vi "exportToDIAdem.vi"(11 "Export Data":string[][](array[string])) -> ()   [LabVIEW 2017]
doc: "This example uses the \"Register ActiveX Event Callback\" with a Microsoft Excel ActiveX control. \nIt demonstrates how to register an event and extract event data."
panel:
  out "Report Path Used":path
  out "Unique Temporary TDR File Path":path
  out "Unique Temporary TDMS File Path":path
  out "error out":errorcluster
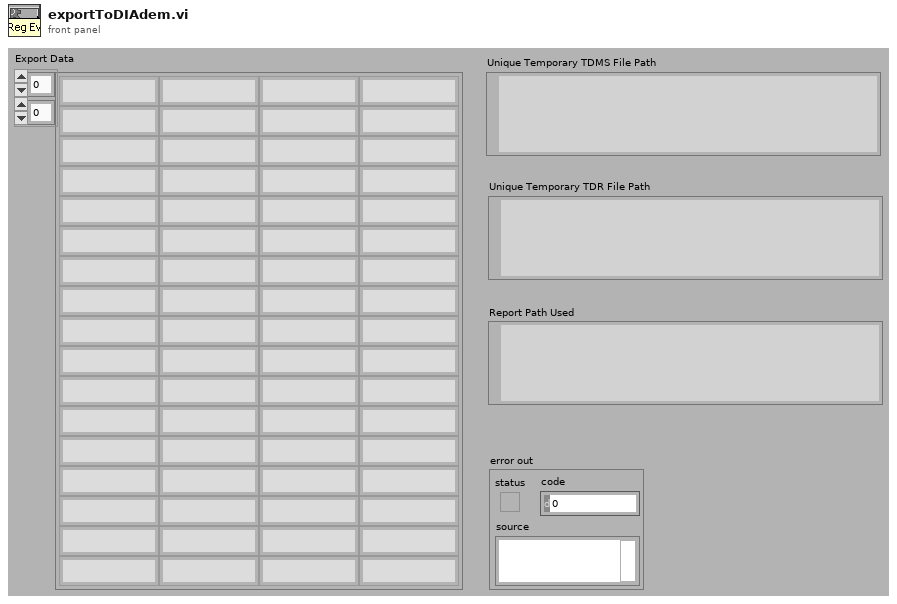
[diagram p1: front panel]
types:
  T1 = enum16{"open", "replace", "create", "open or create", "replace or create", "replace or create with confirmation"}
  T2 = enum16{"open", "open or create", "create or replace", "create", "open (read-only)"}
  T3 = enum32{"invalid app kind", "Development System", "Run Time System", "Student Edition", "Embedded LabVIEW", "Evaluation", "Custom"}
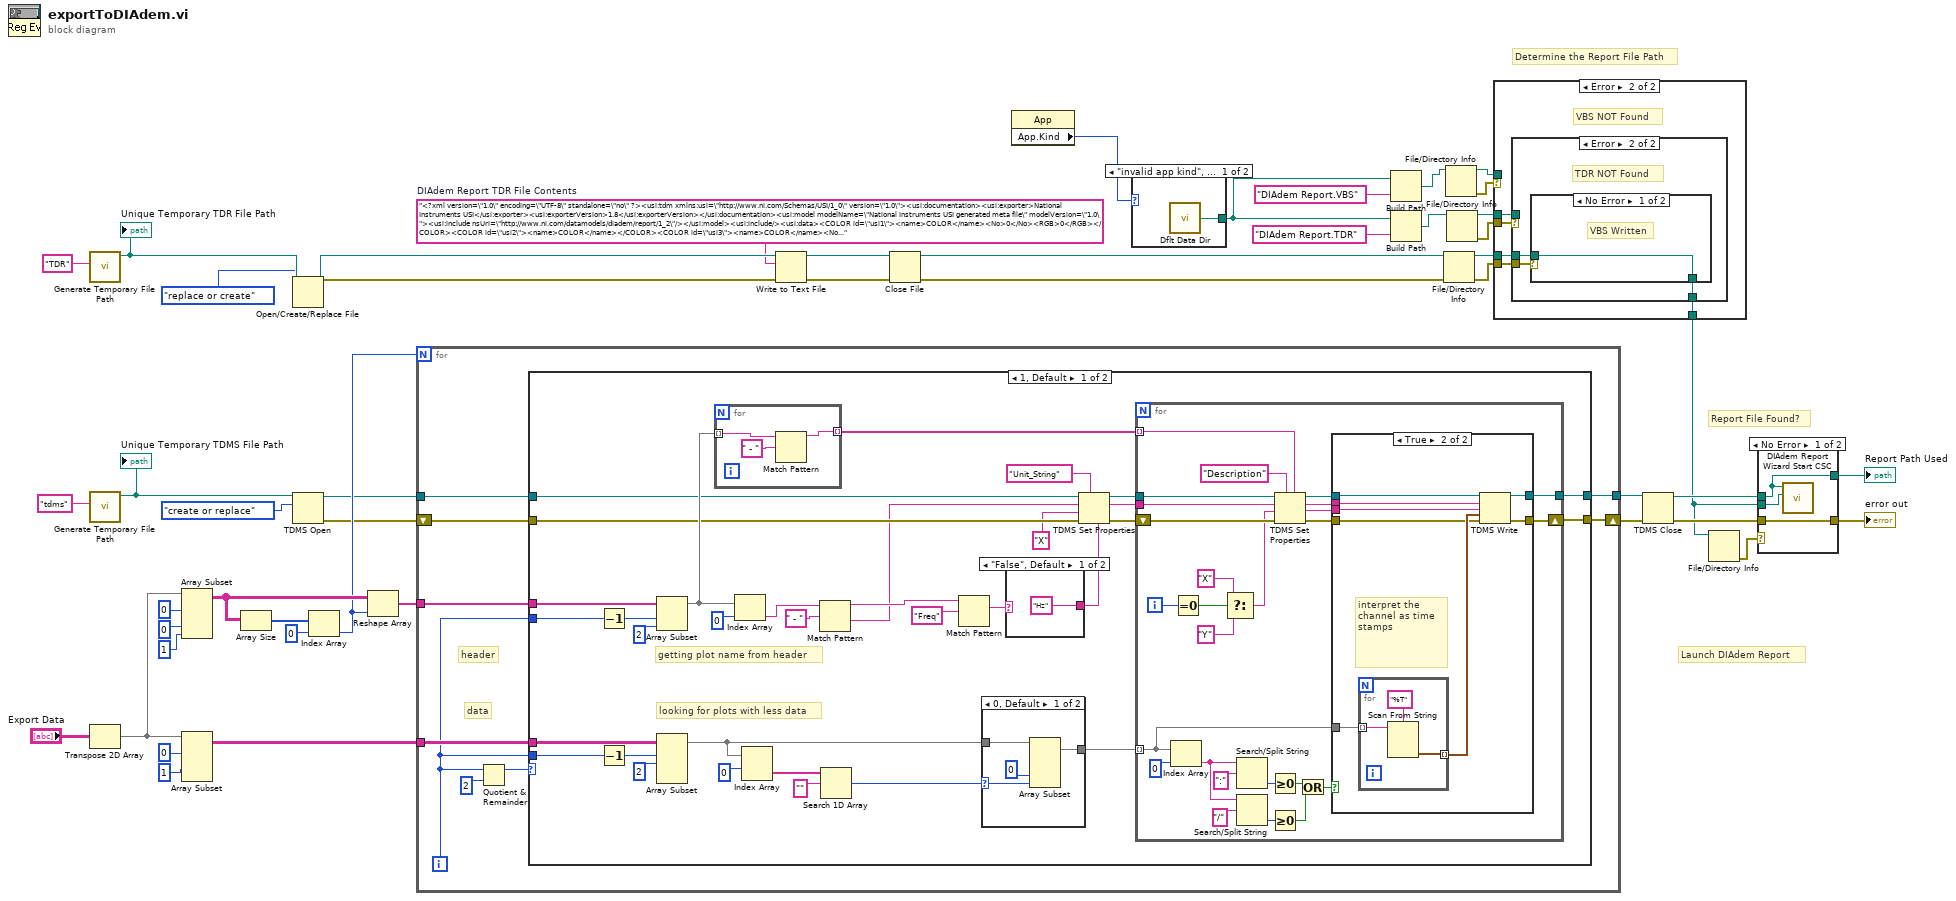
[diagram p0: block diagram]
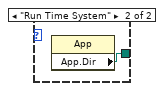
[diagram p2: hidden frame]
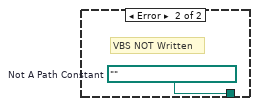
[diagram p5: hidden frame]
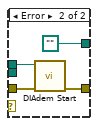
[diagram p6: hidden frame]
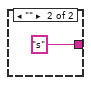
[diagram p7: hidden frame]
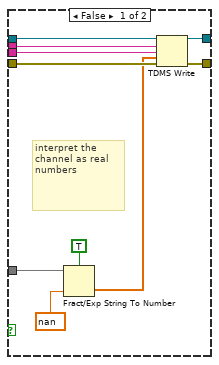
[diagram p8: hidden frame]
diagram:
  w15 = "<?xml version=\"1.0\" encoding=\"UTF-8\" standalone=\"no\" ?><usi:tdm xmlns:usi=\"http://www.ni.com/Schemas/USI/1_0\" version=\"1.0\"><usi:documentation><usi:exporter>National Instruments USI</usi:exporter><usi:exporterVersion>1.8</usi:exporterVersion></usi:documentation><usi:model modelName=\"National Instruments USI generated meta file\" modelVersion=\"1.0\"><usi:include nsUri=\"http://www.ni.com/datamodels/diadem/report/1_2\"/></usi:model><usi:include/><usi:data><COLOR id=\"usi1\"><name>COLOR</name><No>0</No><RGB>0</RGB></COLOR><COLOR id=\"usi2\"><name>COLOR</name></COLOR><COLOR id=\"usi3\"><name>COLOR</name><No>2</No></COLOR><COLOR id=\"usi4\"><name>COLOR</name><No>4</No><RGB>33554687</RGB></COLOR><COLOR id=\"usi5\"><name>COLOR</name><No>3</No><RGB>33619712</RGB></COLOR><COLOR id=\"usi6\"><name>COLOR</name><No>9</No><RGB>50266112</RGB></COLOR><COLOR id=\"usi7\"><name>COLOR</name><No>5</No><RGB>50266367</RGB></COLOR><COLOR id=\"usi8\"><name>COLOR</name><No>6</No><RGB>50331392</RGB></COLOR><COLOR id=\"usi9\"><name>COLOR</name><No>10</No><RGB>46186688</RGB></COLOR><COLOR id=\"usi10\"><name>COLOR</name><No>15</No><RGB>33619967</RGB></COLOR><COLOR id=\"usi11\"><name>COLOR</name><No>9</No><RGB>33554560</RGB></COLOR><COLOR id=\"usi12\"><name>COLOR</name><No>10</No><RGB>33587200</RGB></COLOR><COLOR id=\"usi13\"><name>COLOR</name></COLOR><COLOR id=\"usi14\"><name>COLOR</name></COLOR><COLOR id=\"usi15\"><name>COLOR</name></COLOR><COLOR id=\"usi16\"><name>COLOR</name><No>0</No><RGB>14737616</RGB><RGB2>15263976</RGB2></COLOR><COLOR id=\"usi17\"><name>COLOR</name></COLOR><COLOR id=\"usi18\"><name>COLOR</name></COLOR><COLOR id=\"usi19\"><name>COLOR</name></COLOR><COLOR id=\"usi20\"><name>COLOR</name></COLOR><COLOR id=\"usi21\"><name>COLOR</name></COLOR><COLOR id=\"usi22\"><name>COLOR</name></COLOR><COLOR id=\"usi23\"><name>COLOR</name></COLOR><COLOR id=\"usi24\"><name>COLOR</name></COLOR><COLOR id=\"usi25\"><name>COLOR</name></COLOR><COLOR id=\"usi26\"><name>COLOR</name></COLOR><COLOR id=\"usi27\"><name>COLOR</name></COLOR><COLOR id=\"usi28\"><name>COLOR</name></COLOR><COLOR id=\"usi29\"><name>COLOR</name></COLOR><COLOR id=\"usi30\"><name>COLOR</name><No>2</No><RGB>33554687</RGB></COLOR><COLOR id=\"usi31\"><name>COLOR</name><No>0</No><RGB>50331647</RGB><RGB2>15263976</RGB2></COLOR><COLOR id=\"usi32\"><name>COLOR</name><No>0</No><RGB>0</RGB><RGB2>0</RGB2><FillMode>Horizontal</FillMode></COLOR><COLOR id=\"usi33\"><name>COLOR</name><No>0</No><RGB>0</RGB><RGB2>0</RGB2><FillMode>Horizontal</FillMode></COLOR><COLOR id=\"usi34\"><name>COLOR</name><No>16</No><RGB>50331647</RGB></COLOR><COLOR id=\"usi35\"><name>COLOR</name></COLOR><COLOR id=\"usi36\"><name>COLOR</name><No>0</No><RGB>50331647</RGB></COLOR><COLOR id=\"usi37\"><name>COLOR</name></COLOR><COLOR id=\"usi38\"><name>COLOR</name></COLOR><COLOR id=\"usi39\"><name>COLOR</name></COLOR><COLOR id=\"usi40\"><name>COLOR</name></COLOR><COLOR id=\"usi41\"><name>COLOR</name></COLOR><COLOR id=\"usi42\"><name>COLOR</name><No>7</No><RGB>46186688</RGB></COLOR><COLOR id=\"usi43\"><name>COLOR</name><No>7</No><RGB>46186688</RGB></COLOR><COLOR id=\"usi44\"><name>COLOR</name><No>7</No><RGB>46186688</RGB></COLOR><COLOR id=\"usi45\"><name>COLOR</name><No>7</No><RGB>46186688</RGB></COLOR><COLOR id=\"usi46\"><name>COLOR</name><No>7</No><RGB>46186688</RGB></COLOR><COLOR id=\"usi47\"><name>COLOR</name><No>7</No><RGB>46186688</RGB></COLOR><COLOR id=\"usi48\"><name>COLOR</name><No>7</No><RGB>46186688</RGB></COLOR><COLOR id=\"usi49\"><name>COLOR</name><No>7</No><RGB>46186688</RGB></COLOR><COLOR id=\"usi50\"><name>COLOR</name><No>7</No><RGB>46186688</RGB></COLOR><COLOR id=\"usi51\"><name>COLOR</name><No>7</No><RGB>46186688</RGB></COLOR><COLOR id=\"usi52\"><name>COLOR</name><No>7</No><RGB>46186688</RGB></COLOR><COLOR id=\"usi53\"><name>COLOR</name><No>7</No><RGB>46186688</RGB></COLOR><COLOR id=\"usi54\"><name>COLOR</name><No>7</No><RGB>46186688</RGB></COLOR><COLOR id=\"usi55\"><name>COLOR</name><No>7</No><RGB>46186688</RGB></COLOR><COLOR id=\"usi56\"><name>COLOR</name><No>7</No><RGB>46186688</RGB></COLOR><COLOR id=\"usi57\"><name>COLOR</name><No>7</No><RGB>46186688</RGB></COLOR><COLOR id=\"usi58\"><name>COLOR</name><No>7</No><RGB>46186688</RGB></COLOR><COLOR id=\"usi59\"><name>COLOR</name><No>7</No><RGB>46186688</RGB></COLOR><COLOR id=\"usi60\"><name>COLOR</name><No>7</No><RGB>46186688</RGB></COLOR><COLOR id=\"usi61\"><name>COLOR</name><No>7</No><RGB>46186688</RGB></COLOR><COLOR id=\"usi62\"><name>COLOR</name><RGB>50266112</RGB></COLOR><COLOR id=\"usi63\"><name>COLOR</name></COLOR><COLOR id=\"usi64\"><name>COLOR</name><RGB>50266112</RGB></COLOR><COLOR id=\"usi65\"><name>COLOR</name></COLOR><COLOR id=\"usi66\"><name>COLOR</name><No>2</No><RGB>33554687</RGB></COLOR><COLOR id=\"usi67\"><name>COLOR</name><No>4</No><RGB>50266112</RGB></COLOR><COLOR id=\"usi68\"><name>COLOR</name><No>4</No><RGB>50266112</RGB></COLOR><COLOR id=\"usi69\"><name>COLOR</name><No>2</No><RGB>33554687</RGB></COLOR><COLOR id=\"usi70\"><name>COLOR</name></COLOR><COLOR id=\"usi71\"><name>COLOR</name><No>2</No><RGB>33554687</RGB></COLOR><COLOR id=\"usi72\"><name>COLOR</name></COLOR><COLOR id=\"usi73\"><name>COLOR</name><No>2</No><RGB>33554687</RGB></COLOR><COLOR id=\"usi74\"><name>COLOR</name><No>3</No><RGB>33619712</RGB></COLOR><COLOR id=\"usi75\"><name>COLOR</name><No>4</No><RGB>50266112</RGB></COLOR><COLOR id=\"usi76\"><name>COLOR</name><No>5</No><RGB>50266367</RGB></COLOR><COLOR id=\"usi77\"><name>COLOR</name><No>6</No><RGB>50331392</RGB></COLOR><COLOR id=\"usi78\"><name>COLOR</name><No>7</No><RGB>46186688</RGB></COLOR><COLOR id=\"usi79\"><name>COLOR</name><No>8</No><RGB>33619967</RGB></COLOR><COLOR id=\"usi80\"><name>COLOR</name><No>9</No><RGB>33554560</RGB></COLOR><COLOR id=\"usi81\"><name>COLOR</name><No>10</No><RGB>33587200</RGB></COLOR><COLOR id=\"usi82\"><name>COLOR</name><No>11</No><RGB>41943040</RGB></COLOR><COLOR id=\"usi83\"><name>COLOR</name><No>12</No><RGB>41943168</RGB></COLOR><COLOR id=\"usi84\"><name>COLOR</name><No>13</No><RGB>41975808</RGB></COLOR><COLOR id=\"usi85\"><name>COLOR</name><No>14</No><RGB>41975936</RGB></COLOR><COLOR id=\"usi86\"><name>COLOR</name><No>15</No><RGB>33587328</RGB></COLOR><COLOR id=\"usi87\"><name>COLOR</name><No>4</No><RGB>50266112</RGB></COLOR><COLOR id=\"usi88\"><name>COLOR</name><No>4</No><RGB>50266112</RGB></COLOR><COLOR id=\"usi89\"><name>COLOR</name><No>4</No><RGB>50266112</RGB></COLOR><COLOR id=\"usi90\"><name>COLOR</name><No>4</No><RGB>50266112</RGB></COLOR><LINE id=\"usi91\"><name>FrameLine</name><Width>4</Width><Color>#xpointer(id(\"usi2\"))</Color></LINE><LINE id=\"usi92\"><name>LINE</name><Interval>2</Interval><Width>3</Width><Color>#xpointer(id(\"usi13\"))</Color></LINE><LINE id=\"usi93\"><name>LINE</name><Interval>2</Interval><Width>3</Width><Color>#xpointer(id(\"usi14\"))</Color></LINE><LINE id=\"usi94\"><name>LINE</name><Interval>2</Interval><Width>3</Width><Color>#xpointer(id(\"usi15\"))</Color></LINE><LINE id=\"usi95\"><name>LINE</name><Width>3</Width><Color>#xpointer(id(\"usi27\"))</Color></LINE><LINE id=\"usi96\"><name>LINE</name><Width>3</Width><Color>#xpointer(id(\"usi28\"))</Color></LINE><LINE id=\"usi97\"><name>LINE</name><Width>3</Width><Color>#xpointer(id(\"usi29\"))</Color></LINE><LINE id=\"usi98\"><name>LINE</name><Interval>2</Interval><Width>0</Width><Color>#xpointer(id(\"usi38\"))</Color></LINE><LINE id=\"usi99\"><name>LINE</name><Interval>2</Interval><Width>0</Width><Color>#xpointer(id(\"usi39\"))</Color></LINE><LINE id=\"usi100\"><name>LINE</name><Interval>2</Interval><Width>0</Width><Color>#xpointer(id(\"usi40\"))</Color></LINE><LINE id=\"usi101\"><name>LINE</name><Interval>2</Interval><Width>0</Width><Color>#xpointer(id(\"usi41\"))</Color></LINE><LINE id=\"usi102\"><name>LINE</name><Width>0</Width><Color>#xpointer(id(\"usi67\"))</Color></LINE><FONT id=\"usi103\"><name>FONT</name><Size>3</Size><PitchAndFamily>32</PitchAndFamily><Color>#xpointer(id(\"usi62\"))</Color></FONT><FONT id=\"usi104\"><name>FONT</name><Size>4</Size><PitchAndFamily>16</PitchAndFamily><Color>#xpointer(id(\"usi63\"))</Color></FONT><FONT id=\"usi105\"><name>FONT</name><Size>3</Size><PitchAndFamily>32</PitchAndFamily><Color>#xpointer(id(\"usi64\"))</Color></FONT><FONT id=\"usi106\"><name>FONT</name><Size>4</Size><Angle>90</Angle><PitchAndFamily>16</PitchAndFamily><Color>#xpointer(id(\"usi65\"))</Color></FONT><FONT id=\"usi107\"><name>FONT</name><FaceName>Times New Roman</FaceName><Size>4</Size><PitchAndFamily>16</PitchAndFamily><Color>#xpointer(id(\"usi68\"))</Color></FONT><FONT id=\"usi108\"><name>FONT</name><FaceName>Times New Roman</FaceName><Size>4</Size><PitchAndFamily>16</PitchAndFamily><Color>#xpointer(id(\"usi71\"))</Color></FONT><FONT id=\"usi109\"><name>FONT</name><Size>3</Size><PitchAndFamily>32</PitchAndFamily><Color>#xpointer(id(\"usi87\"))</Color></FONT><FONT id=\"usi110\"><name>FONT</name><Size>3</Size><PitchAndFamily>32</PitchAndFamily><Color>#xpointer(id(\"usi88\"))</Color></FONT><FONT id=\"usi111\"><name>FONT</name><FaceName>Arial</FaceName><Size>3</Size><PitchAndFamily>32</PitchAndFamily><Color>#xpointer(id(\"usi89\"))</Color></FONT><FONT id=\"usi112\"><name>FONT</name><FaceName>Arial</FaceName><Size>3</Size><PitchAndFamily>32</PitchAndFamily><Color>#xpointer(id(\"usi90\"))</Color></FONT><PALETTE2D id=\"usi113\"><Line>#xpointer(id(\"usi213\") id(\"usi214\") id(\"usi215\") id(\"usi216\") id(\"usi217\") id(\"usi218\") id(\"usi219\") id(\"usi220\") id(\"usi221\") id(\"usi222\") id(\"usi223\") id(\"usi224\") id(\"usi225\") id(\"usi226\") id(\"usi227\"))</Line></PALETTE2D><GLOBPAL id=\"usi114\"><name>global Palette 1</name><No>64</No><CtrlColorHSI>7925920 7925760</CtrlColorHSI><Line>#xpointer(id(\"usi92\"))</Line></GLOBPAL><GLOBPAL id=\"usi115\"><name>global Palette 2</name><No>64</No><CtrlColorHSI>7925920 7925999</CtrlColorHSI><Line>#xpointer(id(\"usi93\"))</Line></GLOBPAL><GLOBPAL id=\"usi116\"><name>global Palette 3</name><No>64</No><CtrlColorHSI>11858080 11857920</CtrlColorHSI><Line>#xpointer(id(\"usi94\"))</Line></GLOBPAL><CHANNEL id=\"usi117\"><name>TickChn</name></CHANNEL><CHANNEL id=\"usi118\"><name>TickChn</name></CHANNEL><CHANNEL id=\"usi119\"><name>XChn</name><No>1</No><ChnName>X</ChnName></CHANNEL><CHANNEL id=\"usi120\"><name>YChn</name><No>2</No><ChnName>Y</ChnName></CHANNEL><CHANNEL id=\"usi121\"><name>Y1Chn</name></CHANNEL><CHANNEL id=\"usi122\"><name>CHANNEL</name></CHANNEL><CHANNEL id=\"usi123\"><name>IndexChannel</name></CHANNEL><CHANNEL id=\"usi124\"><name>XChn</name></CHANNEL><CHANNEL id=\"usi125\"><name>YChn</name></CHANNEL><CHANNEL id=\"usi126\"><name>XChn</name></CHANNEL><CHANNEL id=\"usi127\"><name>YChn</name></CHANNEL><CHANNEL id=\"usi128\"><name>XChn</name></CHANNEL><CHANNEL id=\"usi129\"><name>YChn</name></CHANNEL><CHANNEL id=\"usi130\"><name>XChn</name></CHANNEL><CHANNEL id=\"usi131\"><name>YChn</name></CHANNEL><CHANNEL id=\"usi132\"><name>XChn</name></CHANNEL><CHANNEL id=\"usi133\"><name>YChn</name></CHANNEL><CHANNEL id=\"usi134\"><name>XChn</name></CHANNEL><CHANNEL id=\"usi135\"><name>YChn</name></CHANNEL><CHANNEL id=\"usi136\"><name>XChn</name></CHANNEL><CHANNEL id=\"usi137\"><name>YChn</name></CHANNEL><CHANNEL id=\"usi138\"><name>XChn</name></CHANNEL><CHANNEL id=\"usi139\"><name>YChn</name></CHANNEL><CHANNEL id=\"usi140\"><name>XChn</name></CHANNEL><CHANNEL id=\"usi141\"><name>YChn</name></CHANNEL><CHANNEL id=\"usi142\"><name>XChn</name></CHANNEL><CHANNEL id=\"usi143\"><name>YChn</name></CHANNEL><CHANNEL id=\"usi144\"><name>XChn</name></CHANNEL><CHANNEL id=\"usi145\"><name>YChn</name></CHANNEL><CHANNEL id=\"usi146\"><name>XChn</name></CHANNEL><CHANNEL id=\"usi147\"><name>YChn</name></CHANNEL><CHANNEL id=\"usi148\"><name>XChn</name></CHANNEL><CHANNEL id=\"usi149\"><name>YChn</name></CHANNEL><CHANNEL id=\"usi150\"><name>XChn</name></CHANNEL><CHANNEL id=\"usi151\"><name>YChn</name></CHANNEL><CHANNEL id=\"usi152\"><name>XChn</name></CHANNEL><CHANNEL id=\"usi153\"><name>YChn</name></CHANNEL><CHANNEL id=\"usi154\"><name>XChn</name></CHANNEL><CHANNEL id=\"usi155\"><name>YChn</name></CHANNEL><CHANNEL id=\"usi156\"><name>XChn</name></CHANNEL><CHANNEL id=\"usi157\"><name>YChn</name></CHANNEL><CHANNEL id=\"usi158\"><name>XChn</name></CHANNEL><CHANNEL id=\"usi159\"><name>YChn</name></CHANNEL><CHANNEL id=\"usi160\"><name>XChn</name></CHANNEL><CHANNEL id=\"usi161\"><name>YChn</name></CHANNEL><CHANNEL id=\"usi162\"><name>XChn</name></CHANNEL><CHANNEL id=\"usi163\"><name>YChn</name></CHANNEL><CHANNEL id=\"usi164\"><name>PositiveErrorChn</name></CHANNEL><CHANNEL id=\"usi165\"><name>NegativeErrorChn</name></CHANNEL><CHANNEL id=\"usi166\"><name>PositiveErrorChn</name></CHANNEL><CHANNEL id=\"usi167\"><name>NegativeErrorChn</name></CHANNEL><NUMERICLABEL id=\"usi168\"><name>NUMERICLABEL</name><RelPos>bottom</RelPos><Font>#xpointer(id(\"usi103\"))</Font></NUMERICLABEL><NUMERICLABEL id=\"usi169\"><name>NUMERICLABEL</name><RelPos>left</RelPos><Font>#xpointer(id(\"usi105\"))</Font></NUMERICLABEL><FREELABEL id=\"usi170\"><name>FREELABEL</name><Text>@@ChnComment(CurrChnNo)@@ [@@ChnDim(CurrChnNo)@@]</Text><DeltaX>100</DeltaX><DeltaY>-8.07</DeltaY><Font>#xpointer(id(\"usi104\"))</Font></FREELABEL><FREELABEL id=\"usi171\"><name>FREELABEL</name><Text>@@ChnComment(CurrChnNo)@@</Text><DeltaX>-7.51</DeltaX><DeltaY>100</DeltaY><Font>#xpointer(id(\"usi106\"))</Font></FREELABEL><AXISGROUP id=\"usi172\"><name>AxisGroup1</name><XAxis>#xpointer(id(\"usi228\"))</XAxis><YAxis>#xpointer(id(\"usi229\"))</YAxis><AXIS2D>#xpointer(id(\"usi230\"))</AXIS2D></AXISGROUP><PAGE id=\"usi173\"><name>Export From LabVIEW</name><Ratio>0.77</Ratio><Width>10</Width><Height>7.5</Height><PicDefExpand>1</PicDefExpand><Line>#xpointer(id(\"usi91\"))</Line><BackColor>#xpointer(id(\"usi1\"))</BackColor><ExpList>#xpointer(id(\"usi174\"))</ExpList><PalGlob>#xpointer(id(\"usi114\") id(\"usi115\") id(\"usi116\"))</PalGlob><Objects>#xpointer(id(\"usi230\"))</Objects><REPORT>#xpointer(id(\"usi175\"))</REPORT></PAGE><EXPANDLIST id=\"usi174\"><ExpListUse>1</ExpListUse><LineTypUse>0</LineTypUse><LineIntUse>0</LineIntUse><ExpListNo>8</ExpListNo><Line>#xpointer(id(\"usi231\") id(\"usi232\") id(\"usi233\") id(\"usi234\") id(\"usi235\") id(\"usi236\") id(\"usi237\") id(\"usi238\") id(\"usi239\") id(\"usi240\"))</Line></EXPANDLIST><REPORT id=\"usi175\"><name>lvtemporary_550384</name><LastName>lvtemporary_550384</LastName><ScaleNorm>0</ScaleNorm><BinaryRasterOps>13</BinaryRasterOps><Ratio>0.77</Ratio><Width>10</Width><Height>7.5</Height><Pages>#xpointer(id(\"usi173\"))</Pages></REPORT><AXISSYSTEM id=\"usi176\"><FrameDisplay>Frame</FrameDisplay><BackColor>#xpointer(id(\"usi16\"))</BackColor><FrameLine>#xpointer(id(\"usi95\"))</FrameLine><DisplayXAxis>#xpointer(id(\"usi177\"))</DisplayXAxis><DisplayYAxis>#xpointer(id(\"usi178\"))</DisplayYAxis><Sections>#xpointer(id(\"usi179\"))</Sections></AXISSYSTEM><DISPLAYAXIS id=\"usi177\"><GridLine>#xpointer(id(\"usi98\"))</GridLine><MiniTickLine>#xpointer(id(\"usi99\"))</MiniTickLine></DISPLAYAXIS><DISPLAYAXIS id=\"usi178\"><GridLine>#xpointer(id(\"usi100\"))</GridLine><MiniTickLine>#xpointer(id(\"usi101\"))</MiniTickLine></DISPLAYAXIS><SECTIONS id=\"usi179\"><name>Sections</name><Section>#xpointer(id(\"usi180\") id(\"usi181\") id(\"usi182\") id(\"usi183\") id(\"usi184\") id(\"usi185\") id(\"usi186\") id(\"usi187\") id(\"usi188\") id(\"usi189\") id(\"usi190\") id(\"usi191\") id(\"usi192\") id(\"usi193\") id(\"usi194\") id(\"usi195\") id(\"usi196\") id(\"usi197\") id(\"usi198\") id(\"usi199\"))</Section></SECTIONS><SECTION id=\"usi180\"><name>Section1</name><Color>#xpointer(id(\"usi42\"))</Color><XChn>#xpointer(id(\"usi124\"))</XChn><YChn>#xpointer(id(\"usi125\"))</YChn></SECTION><SECTION id=\"usi181\"><name>Section2</name><Color>#xpointer(id(\"usi43\"))</Color><XChn>#xpointer(id(\"usi126\"))</XChn><YChn>#xpointer(id(\"usi127\"))</YChn></SECTION><SECTION id=\"usi182\"><name>Section3</name><Color>#xpointer(id(\"usi44\"))</Color><XChn>#xpointer(id(\"usi128\"))</XChn><YChn>#xpointer(id(\"usi129\"))</YChn></SECTION><SECTION id=\"usi183\"><name>Section4</name><Color>#xpointer(id(\"usi45\"))</Color><XChn>#xpointer(id(\"usi130\"))</XChn><YChn>#xpointer(id(\"usi131\"))</YChn></SECTION><SECTION id=\"usi184\"><name>Section5</name><Color>#xpointer(id(\"usi46\"))</Color><XChn>#xpointer(id(\"usi132\"))</XChn><YChn>#xpointer(id(\"usi133\"))</YChn></SECTION><SECTION id=\"usi185\"><name>Section6</name><Color>#xpointer(id(\"usi47\"))</Color><XChn>#xpointer(id(\"usi134\"))</XChn><YChn>#xpointer(id(\"usi135\"))</YChn></SECTION><SECTION id=\"usi186\"><name>Section7</name><Color>#xpointer(id(\"usi48\"))</Color><XChn>#xpointer(id(\"usi136\"))</XChn><YChn>#xpointer(id(\"usi137\"))</YChn></SECTION><SECTION id=\"usi187\"><name>Section8</name><Color>#xpointer(id(\"usi49\"))</Color><XChn>#xpointer(id(\"usi138\"))</XChn><YChn>#xpointer(id(\"usi139\"))</YChn></SECTION><SECTION id=\"usi188\"><name>Section9</name><Color>#xpointer(id(\"usi50\"))</Color><XChn>#xpointer(id(\"usi140\"))</XChn><YChn>#xpointer(id(\"usi141\"))</YChn></SECTION><SECTION id=\"usi189\"><name>Section10</name><Color>#xpointer(id(\"usi51\"))</Color><XChn>#xpointer(id(\"usi142\"))</XChn><YChn>#xpointer(id(\"usi143\"))</YChn></SECTION><SECTION id=\"usi190\"><name>Section11</name><Color>#xpointer(id(\"usi52\"))</Color><XChn>#xpointer(id(\"usi144\"))</XChn><YChn>#xpointer(id(\"usi145\"))</YChn></SECTION><SECTION id=\"usi191\"><name>Section12</name><Color>#xpointer(id(\"usi53\"))</Color><XChn>#xpointer(id(\"usi146\"))</XChn><YChn>#xpointer(id(\"usi147\"))</YChn></SECTION><SECTION id=\"usi192\"><name>Section13</name><Color>#xpointer(id(\"usi54\"))</Color><XChn>#xpointer(id(\"usi148\"))</XChn><YChn>#xpointer(id(\"usi149\"))</YChn></SECTION><SECTION id=\"usi193\"><name>Section14</name><Color>#xpointer(id(\"usi55\"))</Color><XChn>#xpointer(id(\"usi150\"))</XChn><YChn>#xpointer(id(\"usi151\"))</YChn></SECTION><SECTION id=\"usi194\"><name>Section15</name><Color>#xpointer(id(\"usi56\"))</Color><XChn>#xpointer(id(\"usi152\"))</XChn><YChn>#xpointer(id(\"usi153\"))</YChn></SECTION><SECTION id=\"usi195\"><name>Section16</name><Color>#xpointer(id(\"usi57\"))</Color><XChn>#xpointer(id(\"usi154\"))</XChn><YChn>#xpointer(id(\"usi155\"))</YChn></SECTION><SECTION id=\"usi196\"><name>Section17</name><Color>#xpointer(id(\"usi58\"))</Color><XChn>#xpointer(id(\"usi156\"))</XChn><YChn>#xpointer(id(\"usi157\"))</YChn></SECTION><SECTION id=\"usi197\"><name>Section18</name><Color>#xpointer(id(\"usi59\"))</Color><XChn>#xpointer(id(\"usi158\"))</XChn><YChn>#xpointer(id(\"usi159\"))</YChn></SECTION><SECTION id=\"usi198\"><name>Section19</name><Color>#xpointer(id(\"usi60\"))</Color><XChn>#xpointer(id(\"usi160\"))</XChn><YChn>#xpointer(id(\"usi161\"))</YChn></SECTION><SECTION id=\"usi199\"><name>Section20</name><Color>#xpointer(id(\"usi61\"))</Color><XChn>#xpointer(id(\"usi162\"))</XChn><YChn>#xpointer(id(\"usi163\"))</YChn></SECTION><CURVE2D id=\"usi200\"><name>2DAxis1_Curve1</name><Axis>#xpointer(id(\"usi172\"))</Axis><XChn>#xpointer(id(\"usi119\"))</XChn><YChn>#xpointer(id(\"usi120\"))</YChn><Y1Chn>#xpointer(id(\"usi121\"))</Y1Chn><Line>#xpointer(id(\"usi241\"))</Line><Bar>#xpointer(id(\"usi201\"))</Bar><Symbol>#xpointer(id(\"usi255\"))</Symbol><Marker>#xpointer(id(\"usi205\"))</Marker><ErrorBar>#xpointer(id(\"usi204\"))</ErrorBar><EndLabel>#xpointer(id(\"usi206\"))</EndLabel><Palette>#xpointer(id(\"usi113\"))</Palette><AXIS2D>#xpointer(id(\"usi230\"))</AXIS2D></CURVE2D><BAR2D id=\"usi201\"><Line>#xpointer(id(\"usi252\"))</Line><Filling>#xpointer(id(\"usi102\"))</Filling></BAR2D><ERRORBAR id=\"usi202\"><name>ErrorBar</name><AbsoluteErrorValue>1</AbsoluteErrorValue><PercentageErrorValue>5</PercentageErrorValue><PositiveErrorChn>#xpointer(id(\"usi164\"))</PositiveErrorChn><NegativeErrorChn>#xpointer(id(\"usi165\"))</NegativeErrorChn></ERRORBAR><ERRORBAR id=\"usi203\"><name>ErrorBar</name><AbsoluteErrorValue>1</AbsoluteErrorValue><PercentageErrorValue>5</PercentageErrorValue><PositiveErrorChn>#xpointer(id(\"usi166\"))</PositiveErrorChn><NegativeErrorChn>#xpointer(id(\"usi167\"))</NegativeErrorChn></ERRORBAR><ERRORBAR2D id=\"usi204\"><Line>#xpointer(id(\"usi254\"))</Line><XErrorBar>#xpointer(id(\"usi202\"))</XErrorBar><YErrorBar>#xpointer(id(\"usi203\"))</YErrorBar></ERRORBAR2D><MARK2D id=\"usi205\"><OutLine>#xpointer(id(\"usi253\"))</OutLine><Filling>#xpointer(id(\"usi266\"))</Filling></MARK2D><ENDLABEL id=\"usi206\"><name>EndLabel</name><ConstPos>largest value</ConstPos><Font>#xpointer(id(\"usi108\"))</Font><BackColor>#xpointer(id(\"usi33\"))</BackColor></ENDLABEL><CURVELEGEND id=\"usi207\"><Body>#xpointer(id(\"usi208\"))</Body><Frame>#xpointer(id(\"usi267\"))</Frame><Title>#xpointer(id(\"usi210\"))</Title><Label>#xpointer(id(\"usi269\"))</Label></CURVELEGEND><LEGENDBODY id=\"usi208\"><Draw>1</Draw><PosX>79.67</PosX><PosY>95.9</PosY><RelPos>top left</RelPos><MoveType>only with axis system</MoveType><SizeGlobalX>18.85</SizeGlobalX><SizeGlobalY>83.6</SizeGlobalY><SizeLocalX>20</SizeLocalX><Orientation>vertical</Orientation><BackColor>#xpointer(id(\"usi34\"))</BackColor></LEGENDBODY><LEGENDBODY id=\"usi209\"><PosX>67.86</PosX><PosY>10</PosY><BackColor>#xpointer(id(\"usi36\"))</BackColor></LEGENDBODY><TITLE id=\"usi210\"><name>Title</name><Font>#xpointer(id(\"usi109\"))</Font></TITLE><TITLE id=\"usi211\"><name>Title</name><Font>#xpointer(id(\"usi111\"))</Font></TITLE><COLORLEGEND id=\"usi212\"><Body>#xpointer(id(\"usi209\"))</Body><Frame>#xpointer(id(\"usi268\"))</Frame><Title>#xpointer(id(\"usi211\"))</Title><Label>#xpointer(id(\"usi270\"))</Label></COLORLEGEND><PALLINE id=\"usi213\"><name>PALLINE[1]</name><Interval>5</Interval><Width>0</Width><Color>#xpointer(id(\"usi72\"))</Color></PALLINE><PALLINE id=\"usi214\"><name>PALLINE[2]</name><Interval>5</Interval><Width>0</Width><Color>#xpointer(id(\"usi73\"))</Color></PALLINE><PALLINE id=\"usi215\"><name>PALLINE[3]</name><Interval>5</Interval><Width>0</Width><Color>#xpointer(id(\"usi74\"))</Color></PALLINE><PALLINE id=\"usi216\"><name>PALLINE[4]</name><Interval>5</Interval><Width>0</Width><Color>#xpointer(id(\"usi75\"))</Color></PALLINE><PALLINE id=\"usi217\"><name>PALLINE[5]</name><Interval>5</Interval><Width>0</Width><Color>#xpointer(id(\"usi76\"))</Color></PALLINE><PALLINE id=\"usi218\"><name>PALLINE[6]</name><Interval>5</Interval><Width>0</Width><Color>#xpointer(id(\"usi77\"))</Color></PALLINE><PALLINE id=\"usi219\"><name>PALLINE[7]</name><Interval>5</Interval><Width>0</Width><Color>#xpointer(id(\"usi78\"))</Color></PALLINE><PALLINE id=\"usi220\"><name>PALLINE[8]</name><Interval>5</Interval><Width>0</Width><Color>#xpointer(id(\"usi79\"))</Color></PALLINE><PALLINE id=\"usi221\"><name>PALLINE[9]</name><Interval>5</Interval><Width>0</Width><Color>#xpointer(id(\"usi80\"))</Color></PALLINE><PALLINE id=\"usi222\"><name>PALLINE[10]</name><Interval>5</Interval><Width>0</Width><Color>#xpointer(id(\"usi81\"))</Color></PALLINE><PALLINE id=\"usi223\"><name>PALLINE[11]</name><Interval>5</Interval><Width>0</Width><Color>#xpointer(id(\"usi82\"))</Color></PALLINE><PALLINE id=\"usi224\"><name>PALLINE[12]</name><Interval>5</Interval><Width>0</Width><Color>#xpointer(id(\"usi83\"))</Color></PALLINE><PALLINE id=\"usi225\"><name>PALLINE[13]</name><Interval>5</Interval><Width>0</Width><Color>#xpointer(id(\"usi84\"))</Color></PALLINE><PALLINE id=\"usi226\"><name>PALLINE[14]</name><Interval>5</Interval><Width>0</Width><Color>#xpointer(id(\"usi85\"))</Color></PALLINE><PALLINE id=\"usi227\"><name>PALLINE[15]</name><Interval>5</Interval><Width>0</Width><Color>#xpointer(id(\"usi86\"))</Color></PALLINE><XAXIS2D id=\"usi228\"><name>2DAxis1_XAxis1</name><BeginValue>63079603200</BeginValue><EndValue>63142761600</EndValue><SpanWidth>63158400</SpanWidth><Origin>63079603200</Origin><TickDistance>7776000</TickDistance><MiniTick>2</MiniTick><DivMode>Date/Time</DivMode><OffsetOrigin>AxisBegin</OffsetOrigin><TickType>bottom</TickType><ScaleInUnits>1</ScaleInUnits><AutoScaleUnits>1</AutoScaleUnits><TickChn>#xpointer(id(\"usi117\"))</TickChn><Line>#xpointer(id(\"usi96\"))</Line><NumericLabel>#xpointer(id(\"usi168\"))</NumericLabel><FreeLabel>#xpointer(id(\"usi170\"))</FreeLabel></XAXIS2D><YAXIS2D id=\"usi229\"><name>2DAxis1_YAxis1</name><BeginValue>-11</BeginValue><EndValue>32</EndValue><SpanWidth>43</SpanWidth><TickDistance>10</TickDistance><OffsetOrigin>AxisBegin</OffsetOrigin><Heigth>100</Heigth><TickType>left</TickType><ScaleInUnits>1</ScaleInUnits><AutoScaleUnits>1</AutoScaleUnits><TickChn>#xpointer(id(\"usi118\"))</TickChn><Line>#xpointer(id(\"usi97\"))</Line><NumericLabel>#xpointer(id(\"usi169\"))</NumericLabel><FreeLabel>#xpointer(id(\"usi171\"))</FreeLabel></YAXIS2D><AXIS2D id=\"usi230\"><name>2DAxis1</name><LastName>2DAxis1</LastName><left>11.52</left><right>20.7</right><top>4.1</top><bottom>12.3</bottom><ScaledSize>3 3</ScaledSize><PAGE>#xpointer(id(\"usi173\"))</PAGE><AxisSystem>#xpointer(id(\"usi176\"))</AxisSystem><XAxes>#xpointer(id(\"usi228\"))</XAxes><YAxes>#xpointer(id(\"usi229\"))</YAxes><Axes>#xpointer(id(\"usi172\"))</Axes><Curves>#xpointer(id(\"usi200\"))</Curves><CurveLegend>#xpointer(id(\"usi207\"))</CurveLegend><ColorLegend>#xpointer(id(\"usi212\"))</ColorLegend></AXIS2D><EXPANDLINE id=\"usi231\"><name>Line 1</name><Interval>2</Interval><Width>3</Width><Color>#xpointer(id(\"usi3\"))</Color><OutLine>#xpointer(id(\"usi242\"))</OutLine><Filling>#xpointer(id(\"usi256\"))</Filling></EXPANDLINE><EXPANDLINE id=\"usi232\"><name>Line 2</name><Interval>2</Interval><Width>3</Width><Color>#xpointer(id(\"usi4\"))</Color><OutLine>#xpointer(id(\"usi243\"))</OutLine><Filling>#xpointer(id(\"usi257\"))</Filling></EXPANDLINE><EXPANDLINE id=\"usi233\"><name>Line 3</name><Interval>2</Interval><Width>3</Width><Color>#xpointer(id(\"usi5\"))</Color><OutLine>#xpointer(id(\"usi244\"))</OutLine><Filling>#xpointer(id(\"usi258\"))</Filling></EXPANDLINE><EXPANDLINE id=\"usi234\"><name>Line 4</name><Interval>2</Interval><Width>3</Width><Color>#xpointer(id(\"usi6\"))</Color><OutLine>#xpointer(id(\"usi245\"))</OutLine><Filling>#xpointer(id(\"usi259\"))</Filling></EXPANDLINE><EXPANDLINE id=\"usi235\"><name>Line 5</name><Interval>2</Interval><Width>3</Width><Color>#xpointer(id(\"usi7\"))</Color><OutLine>#xpointer(id(\"usi246\"))</OutLine><Filling>#xpointer(id(\"usi260\"))</Filling></EXPANDLINE><EXPANDLINE id=\"usi236\"><name>Line 6</name><Interval>2</Interval><Width>3</Width><Color>#xpointer(id(\"usi8\"))</Color><OutLine>#xpointer(id(\"usi247\"))</OutLine><Filling>#xpointer(id(\"usi261\"))</Filling></EXPANDLINE><EXPANDLINE id=\"usi237\"><name>Line 7</name><Interval>2</Interval><Width>3</Width><Color>#xpointer(id(\"usi9\"))</Color><OutLine>#xpointer(id(\"usi248\"))</OutLine><Filling>#xpointer(id(\"usi262\"))</Filling></EXPANDLINE><EXPANDLINE id=\"usi238\"><name>Line 8</name><Interval>2</Interval><Width>3</Width><Color>#xpointer(id(\"usi10\"))</Color><OutLine>#xpointer(id(\"usi249\"))</OutLine><Filling>#xpointer(id(\"usi263\"))</Filling></EXPANDLINE><EXPANDLINE id=\"usi239\"><name>Line 9</name><Interval>2</Interval><Width>0</Width><Color>#xpointer(id(\"usi11\"))</Color><OutLine>#xpointer(id(\"usi250\"))</OutLine><Filling>#xpointer(id(\"usi264\"))</Filling></EXPANDLINE><EXPANDLINE id=\"usi240\"><name>Line 10</name><Interval>2</Interval><Width>0</Width><Color>#xpointer(id(\"usi12\"))</Color><OutLine>#xpointer(id(\"usi251\"))</OutLine><Filling>#xpointer(id(\"usi265\"))</Filling></EXPANDLINE><LINE2D id=\"usi241\"><name>LINE2D</name><Interval>5</Interval><Width>2</Width><Color>#xpointer(id(\"usi30\"))</Color><FillColor>#xpointer(id(\"usi31\"))</FillColor></LINE2D><BARLINE id=\"usi242\"><name>BARLINE</name><Width>0</Width><Color>#xpointer(id(\"usi17\"))</Color></BARLINE><BARLINE id=\"usi243\"><name>BARLINE</name><Width>0</Width><Color>#xpointer(id(\"usi18\"))</Color></BARLINE><BARLINE id=\"usi244\"><name>BARLINE</name><Width>0</Width><Color>#xpointer(id(\"usi19\"))</Color></BARLINE><BARLINE id=\"usi245\"><name>BARLINE</name><Width>0</Width><Color>#xpointer(id(\"usi20\"))</Color></BARLINE><BARLINE id=\"usi246\"><name>BARLINE</name><Width>0</Width><Color>#xpointer(id(\"usi21\"))</Color></BARLINE><BARLINE id=\"usi247\"><name>BARLINE</name><Width>0</Width><Color>#xpointer(id(\"usi22\"))</Color></BARLINE><BARLINE id=\"usi248\"><name>BARLINE</name><Width>0</Width><Color>#xpointer(id(\"usi23\"))</Color></BARLINE><BARLINE id=\"usi249\"><name>BARLINE</name><Width>0</Width><Color>#xpointer(id(\"usi24\"))</Color></BARLINE><BARLINE id=\"usi250\"><name>BARLINE</name><Width>0</Width><Color>#xpointer(id(\"usi25\"))</Color></BARLINE><BARLINE id=\"usi251\"><name>BARLINE</name><Width>0</Width><Color>#xpointer(id(\"usi26\"))</Color></BARLINE><BARLINE id=\"usi252\"><name>BarLine</name><Interval>5</Interval><Width>0</Width><Color>#xpointer(id(\"usi66\"))</Color></BARLINE><BARLINE id=\"usi253\"><name>BARLINE</name><Width>0</Width><AutoColor>1</AutoColor><Color>#xpointer(id(\"usi69\"))</Color></BARLINE><ERRORBARLINE id=\"usi254\"><name>LINE</name><Interval>5</Interval><Width>0</Width><Color>#xpointer(id(\"usi70\"))</Color></ERRORBARLINE><SYMBOL2D id=\"usi255\"><name>SYMBOL2D</name><XNumFormat></XNumFormat><PointNumFormat></PointNumFormat><ChnNumFormat></ChnNumFormat><Separator>Blank</Separator><Channel>#xpointer(id(\"usi122\"))</Channel><IndexChannel>#xpointer(id(\"usi123\"))</IndexChannel><Font>#xpointer(id(\"usi107\"))</Font><BackColor>#xpointer(id(\"usi32\"))</BackColor></SYMBOL2D><FILLING id=\"usi256\"><name>Filling</name></FILLING><FILLING id=\"usi257\"><name>Filling</name></FILLING><FILLING id=\"usi258\"><name>Filling</name></FILLING><FILLING id=\"usi259\"><name>Filling</name></FILLING><FILLING id=\"usi260\"><name>Filling</name></FILLING><FILLING id=\"usi261\"><name>Filling</name></FILLING><FILLING id=\"usi262\"><name>Filling</name></FILLING><FILLING id=\"usi263\"><name>Filling</name></FILLING><FILLING id=\"usi264\"><name>Filling</name></FILLING><FILLING id=\"usi265\"><name>Filling</name></FILLING><FILLING id=\"usi266\"><name>Filling</name><No>0</No><RGB>46186688</RGB></FILLING><FRAME id=\"usi267\"><name>FRAME</name><Width>3</Width><Draw>1</Draw><Color>#xpointer(id(\"usi35\"))</Color></FRAME><FRAME id=\"usi268\"><name>FRAME</name><Width>3</Width><Draw>1</Draw><Color>#xpointer(id(\"usi37\"))</Color></FRAME><CURVELEGENDLABEL id=\"usi269\"><name>CURVELEGENDLABEL</name><Size>15</Size><TextSizeAuto>1</TextSizeAuto><TextColorAuto>1</TextColorAuto><TextType>ChannelGroup</TextType><RelWidth>1</RelWidth><Font>#xpointer(id(\"usi110\"))</Font></CURVELEGENDLABEL><COLORLEGENDLABEL id=\"usi270\"><name>COLORLEGENDLABEL</name><Size>30</Size><TextSizeAuto>1</TextSizeAuto><Font>#xpointer(id(\"usi112\"))</Font></COLORLEGENDLABEL></usi:data></usi:tdm>"  # DIAdem Report TDR File Contents
  # "Determine the Report File Path"
  # "Report File Found?"
  # "Launch DIAdem Report"
  n1 = call <vilib>:"Generate Temporary File Path.vi"("Temporary File Extension (tmp)"="TDR") -> ("Unique Temporary File Path"=w21:path)  [unwired: 9 in, 1 out]
  "Unique Temporary TDR File Path" <- w21
  n2 = call <vilib>:"Generate Temporary File Path.vi"("Temporary File Extension (tmp)"="tdms") -> ("Unique Temporary File Path"=w30:path)  [unwired: 9 in, 1 out]
  "Unique Temporary TDMS File Path" <- w30
  n3 = Transpose 2D Array(2D array="Export Data") -> (transposed array=w25:string[][])
  n4 = Array Subset(array=w25, index (row)=0 ("index"), index (col)=0 ("index"), length (col)=1 ("length")) -> (w41:string[][])  [unwired: 1 in]
  n5 = Array Subset(array=w25, index (row)=0 ("index"), index (col)=1 ("index")) -> (w37:string[][])  [unwired: 2 in]
  n6 = Array Size(array=w41) -> (size(s)=w40:i32[])
  n7 = Open/Create/Replace File(file path (use dialog)=w21, operation (0:open)=T1."replace or create") -> (refnum out=w19:refnum<file>, error out=w17:errorcluster)  [unwired: 4 in, 1 out]
  n8 = TDMS Open(10:T2."create or replace" ("operation (0:open)"), 11:w30) -> (0:w31:errorcluster, 3:w32:refnum<k34>)  [unwired: 5 in]
  n9 = Index Array(array=w40, index=0) -> (element=w33:i32)
  n10 = Reshape Array(w41, w33) -> (w38:string[])
  n11 = for {
    N: w33 -> [_]
    tunnel: w32 -> [w54]
    shift-right: [w55] -> w35
    shift-left: w31 -> [w53]
    tunnel: [w52] -> w34
    tunnel: w37 -> [w51]
    tunnel: w38 -> [w56]
    i -> [w50]
    # "data"
    # "header"
    n12 = Quotient & Remainder(x=w50, y=2) -> (x-y*floor(x/y)=w49:i32)  [unwired: 1 out]
    n13 = case shown="1, Default" w49 {
      tunnel: w56 -> [w71 _]
      tunnel: w50 -> [w88 _]
      tunnel: w50 -> [w86 _]
      tunnel: [w76 w149] -> w55
      tunnel: w54 -> [w65 w148]
      tunnel: w53 -> [w64 w149]
      tunnel: [w75 w148] -> w52
      tunnel: w51 -> [w74 _]
      frame 1, Default {
        # "getting plot name from header"
        # "looking for plots with less data"
        n14 = Decrement(x=w88) -> (x-1=w87:i32)
        n15 = Decrement(x=w86) -> (x-1=w85:i32)
        n16 = Array Subset(array=w71, index=w87, length=2) -> (w73:string[])
        n17 = Array Subset(array=w74, index (row)=w85, length (row)=2 ("length")) -> (w78:string[][])  [unwired: 2 in]
        n18 = for {
          tunnel: w73 -> [w94] mode=indexing
          tunnel: [w93] -> w72 mode=indexing
          n19 = Match Pattern(string=w94, regular expression=" - ") -> (before substring=w93:string)  [unwired: 1 in, 3 out]
        }
        n20 = Index Array(array=w73, index=0) -> (element=w82:string)
        n21 = Index Array(array=w78, index (row)=0 ("index")) -> (element=w80:string[])  [unwired: 1 in]
        n22 = Match Pattern(string=w82, regular expression=" - ") -> (before substring=w60:string, after substring=w59:string)  [unwired: 1 in, 2 out]
        n23 = Search 1D Array(1D array=w80, element="") -> (index of element=w62:i32)  [unwired: 1 in]
        n24 = Match Pattern(string=w60, regular expression="Freq") -> (match substring=w61:string)  [unwired: 1 in, 3 out]
        n25 = case shown="0, Default" w62 {
          selector: w62 -> [w143 _]
          tunnel: [w145 w147] -> w77
          tunnel: w78 -> [w144 w147]
          frame 0, Default {
            n26 = Array Subset(array=w144, index (col)=0 ("index"), length (col)=w143) -> (w145:string[][])  [unwired: 2 in]
          }
          frame -1 {
          }
        }
        n27 = case shown="\"False\", Default" w61 {
          tunnel: ["Hz" "s" ("format string")] -> w68
          frame "False", Default {
          }
          frame "" {
          }
        }
        n28 = TDMS Set Properties(5:w68, 7:"Unit_String" ("format string"), 8:w64, 9:"X" ("format string"), 10:w59, 11:w65) -> (0:w63:errorcluster, 2:w66:string, 3:w67:refnum<k34>)  [unwired: 1 out]
        n29 = for {
          tunnel: w77 -> [w119] mode=indexing
          tunnel: w67 -> [w97]
          tunnel: w72 -> [w102] mode=indexing
          shift-right: [w121] -> w76
          shift-left: w63 -> [w105]
          tunnel: [w120] -> w75
          tunnel: w66 -> [w103]
          i -> [w109]
          n30 = Index Array(array=w119, index=0) -> (element=w115:string)
          n31 = Equal To 0?(x=w109) -> (x = 0?=w108:bool)
          n32 = Select(t="X" ("format string"), s=w108, f="Y" ("format string")) -> (s? t:f=w99:string)
          n33 = Search/Split String(string=w115, search string/char (-)=":") -> (offset of match=w113:i32)  [unwired: 1 in, 2 out]
          n34 = Search/Split String(string=w115, search string/char (-)="/") -> (offset of match=w114:i32)  [unwired: 1 in, 2 out]
          n35 = Greater Or Equal To 0?(x=w113) -> (x >= 0?=w111:bool)
          n36 = Greater Or Equal To 0?(x=w114) -> (x >= 0?=w110:bool)
          n37 = TDMS Set Properties(5:w102, 7:"Description" ("format string"), 8:w105, 9:w99, 10:w103, 11:w97) -> (0:w104:errorcluster, 1:w98:string, 2:w100:string, 3:w96:refnum<k34>)
          n38 = Or(x=w111, y=w110) -> (x .or. y?=w112:bool)
          n39 = case shown="True" w112 {
            tunnel: w96 -> [w129 w135]
            tunnel: w100 -> [w128 w133]
            tunnel: w98 -> [w127 w134]
            tunnel: [w131 w139] -> w121
            tunnel: [w130 w138] -> w120
            tunnel: w104 -> [w126 w132]
            tunnel: w119 -> [w124 w137]
            frame False {
              # "interpret the channel as real numbers"
              n40 = Fract/Exp String To Number(use system decimal point (T)=TRUE, string=w124, default (0 dbl)=nan) -> (number=w123:dbl[])  [unwired: 1 in, 1 out]
              n41 = TDMS Write(0:w129, 5:w128, 7:w127, 9:w123, 11:w126) -> (4:w130:refnum<k34>, 15:w131:errorcluster)  [unwired: 1 in, 2 out]
            }
            frame True {
              # "interpret the channel as time stamps"
              n42 = for {
                tunnel: w137 -> [w140] mode=indexing
                tunnel: [w141] -> w136 mode=indexing
                n43 = Scan From String(format string="%T", input string=w140) -> (output 1=w141:timestamp)  [unwired: 3 in, 3 out]
              }
              n44 = TDMS Write(0:w135, 5:w133, 7:w134, 9:w136, 11:w132) -> (4:w138:refnum<k34>, 15:w139:errorcluster)  [unwired: 1 in, 2 out]
            }
          }
        }
      }
      frame 0 {
        # "Even iteration (i)"
      }
    }
  }
  n45 = Write to Text File(file (use dialog)=w19, text=w15, error in=w17) -> (refnum out=w18:refnum<file>, error out=w16:errorcluster)  [unwired: 1 in, 1 out]
  n46 = Close File(refnum=w18, error in=w16) -> (path=w6:path, error out=w5:errorcluster)
  n47 = property class="App"() -> ("App.Kind"=w13:T3)  [unwired: 2 in, 2 out]
  n48 = case shown="\"invalid app kind\", Default" w13 {
    tunnel: [w150 w151] -> w24
    frame "invalid app kind", Default {
      n49 = call <vilib>:"Dflt Data Dir.vi"() -> ("App:Default Data Directory"=w150:path)
    }
    frame "Run Time System" {
      n50 = property class="App"() -> ("App.Dir"=w151:path)  [unwired: 2 in, 2 out]
    }
  }
  n51 = Build Path(base path=w24, name or relative path="DIAdem Report.VBS") -> (appended path=w12:path)
  n52 = Build Path(base path=w24, name or relative path="DIAdem Report.TDR") -> (appended path=w9:path)
  n53 = File/Directory Info(path=w6, error in=w5) -> (path out=w4:path, error out=w3:errorcluster)  [unwired: 5 out]
  n54 = File/Directory Info(path=w12) -> (path out=w11:path, error out=w10:errorcluster)  [unwired: 1 in, 5 out]
  n55 = File/Directory Info(path=w9) -> (path out=w8:path, error out=w7:errorcluster)  [unwired: 1 in, 5 out]
  n56 = case shown="Error" w10 {
    tunnel: w11 -> [w152 _]
    tunnel: w8 -> [_ w156]
    tunnel: w7 -> [_ w157]
    tunnel: w4 -> [_ w155]
    tunnel: w3 -> [_ w154]
    tunnel: [w152 w153] -> w2
    frame No Error {
      # "VBS Found"
    }
    frame Error {
      # "VBS NOT Found"
      n57 = case shown="Error" w157 {
        tunnel: w156 -> [w158 _]
        tunnel: w155 -> [_ w159]
        tunnel: w154 -> [_ w161]
        tunnel: [w158 w160] -> w153
        frame No Error {
          # "TDR Found"
        }
        frame Error {
          # "TDR NOT Found"
          n58 = case shown="No Error" w161 {
            tunnel: [w162 w163] -> w160
            tunnel: w159 -> [w162 _]
            frame No Error {
              # "VBS Written"
            }
            frame Error {
              w163 = path ""  # Not A Path Constant
              # "VBS NOT Written"
            }
          }
        }
      }
    }
  }
  n59 = TDMS Close(8:w35, 11:w34) -> (0:w27:errorcluster, 3:w29:path)
  n60 = File/Directory Info(path=w2) -> (error out=w1:errorcluster)  [unwired: 1 in, 6 out]
  n61 = case shown="No Error" w1 {
    tunnel: w2 -> [w164 _]
    tunnel: w29 -> [w165 w170]
    tunnel: [w166 w169] -> w28
    tunnel: w27 -> [w166 w168]
    tunnel: [w165 path "" ("Not A Path Constant")] -> w14
    frame No Error {
      n62 = call <vilib>:"DIAdem Report Wizard Start CSC.vi"("Layout File (Path and File)"=w164, "Data File (Path and File)"=w165) -> ()  [unwired: 5 in, 1 out]
    }
    frame Error {
      n63 = call <vilib>:"DIAdem Start.vi"("error in (no error)"=w168, "Data File (Path and File)"=w170) -> ("error out"=w169:errorcluster)
    }
  }
  "error out" <- w28
  "Report Path Used" <- w14
